vi "Log L16from Y.vi"(8 "error in (no error)":errorcluster, 10 "para1":cluster{}, 11 "para0":dbl) -> (0 "error out":errorcluster, 3 "function return":i32)   [LabVIEW 2018]
doc: "LIBTIFF_DLL_IMPEXP int LogL16fromY(double, int = SGILOGENCODE_NODITHER);"
uses:
  libtiff3.dll
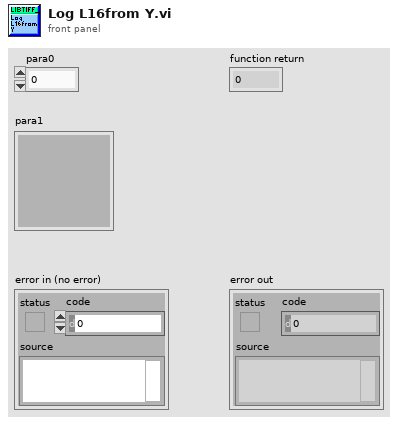
[diagram p1: front panel]
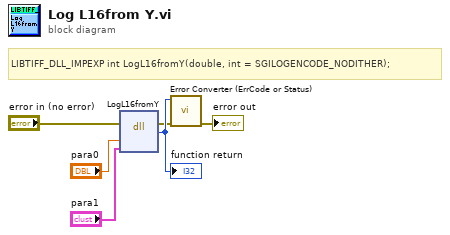
[diagram p0: block diagram]
diagram:
  # "LIBTIFF_DLL_IMPEXP\tint LogL16fromY(double, int = SGILOGENCODE_NODITHER);"
  n1 = dll-call lib="C:/Users/johan/Downloads/LabVIEW software/LabVIEW software/IX-81 Software/lib/tiff/LibTiffLabview/libtiff3.*" fn="LogL16fromY"(error in="error in (no error)", "para0"="para0", "para1"="para1") -> (error out=w2:errorcluster, w6:i32)  [unwired: 4 in, 1 out]
  "function return" <- w6
  n2 = call "Error Converter (ErrCode or Status).vi"("error in (no error)"=w2, "error code"=w6) -> ("error out"=→"error out":errorcluster)  [unwired: 9 in]
